vi "Create Indices.vi"(0 "Standard Engine Configuration":refnum<class "Standard Engine Configuration.lvclass">, 1 "Engine Tags":T1, 5 "main data dictionary":refnum<class "data dictionary.lvclass">, 7 "data description":T5, 9 "Module ID":string, 11 "error in":errorcluster) -> (4 "Input Transfer Specification":T2, 6 "Parameter Transfer Specifcation":T2, 8 "Result Transfer Specifcation":T2, 10 "Output Transfer Specifcation":T2, 15 "error out":errorcluster)   [LabVIEW 2013, in "Standard Engine Runtime.lvclass"]
doc: "Takes a single module's configuration and reformats that into a set of mappings."
uses:
  Standard Engine Runtime.lvclass
  <vilib>/NI/Tag Bus/dictionary/data dictionary.lvclass
  <vilib>/NI/Tag Bus Module Framework/channel/data tables.ctl
  <vilib>/NI/Tag Bus/dictionary table pair.ctl
  <vilib>/NI/Tag Bus/table/data table.ctl
  main engine/module method data.ctl
  <vilib>/NI/Tag Bus/table/transfer specification.ctl
  <vilib>/NI/Tag Bus/tag/Data Type.ctl
  Configuration/Standard Engine Configuration.lvclass
  <vilib>/NI/Module Execution Interface/Engine Configuration/engine configuration.lvclass
  <vilib>/NI/Tag Bus/tag/tag descriptor.lvclass
  <vilib>/NI/Tag Bus/table/data table.lvlib
  main engine/main engine.lvlib
  <vilib>/NI/Tag Bus Module Framework/channel/TBM channel.lvclass
  <vilib>/NI/Tag Bus/tag bus.lvlib
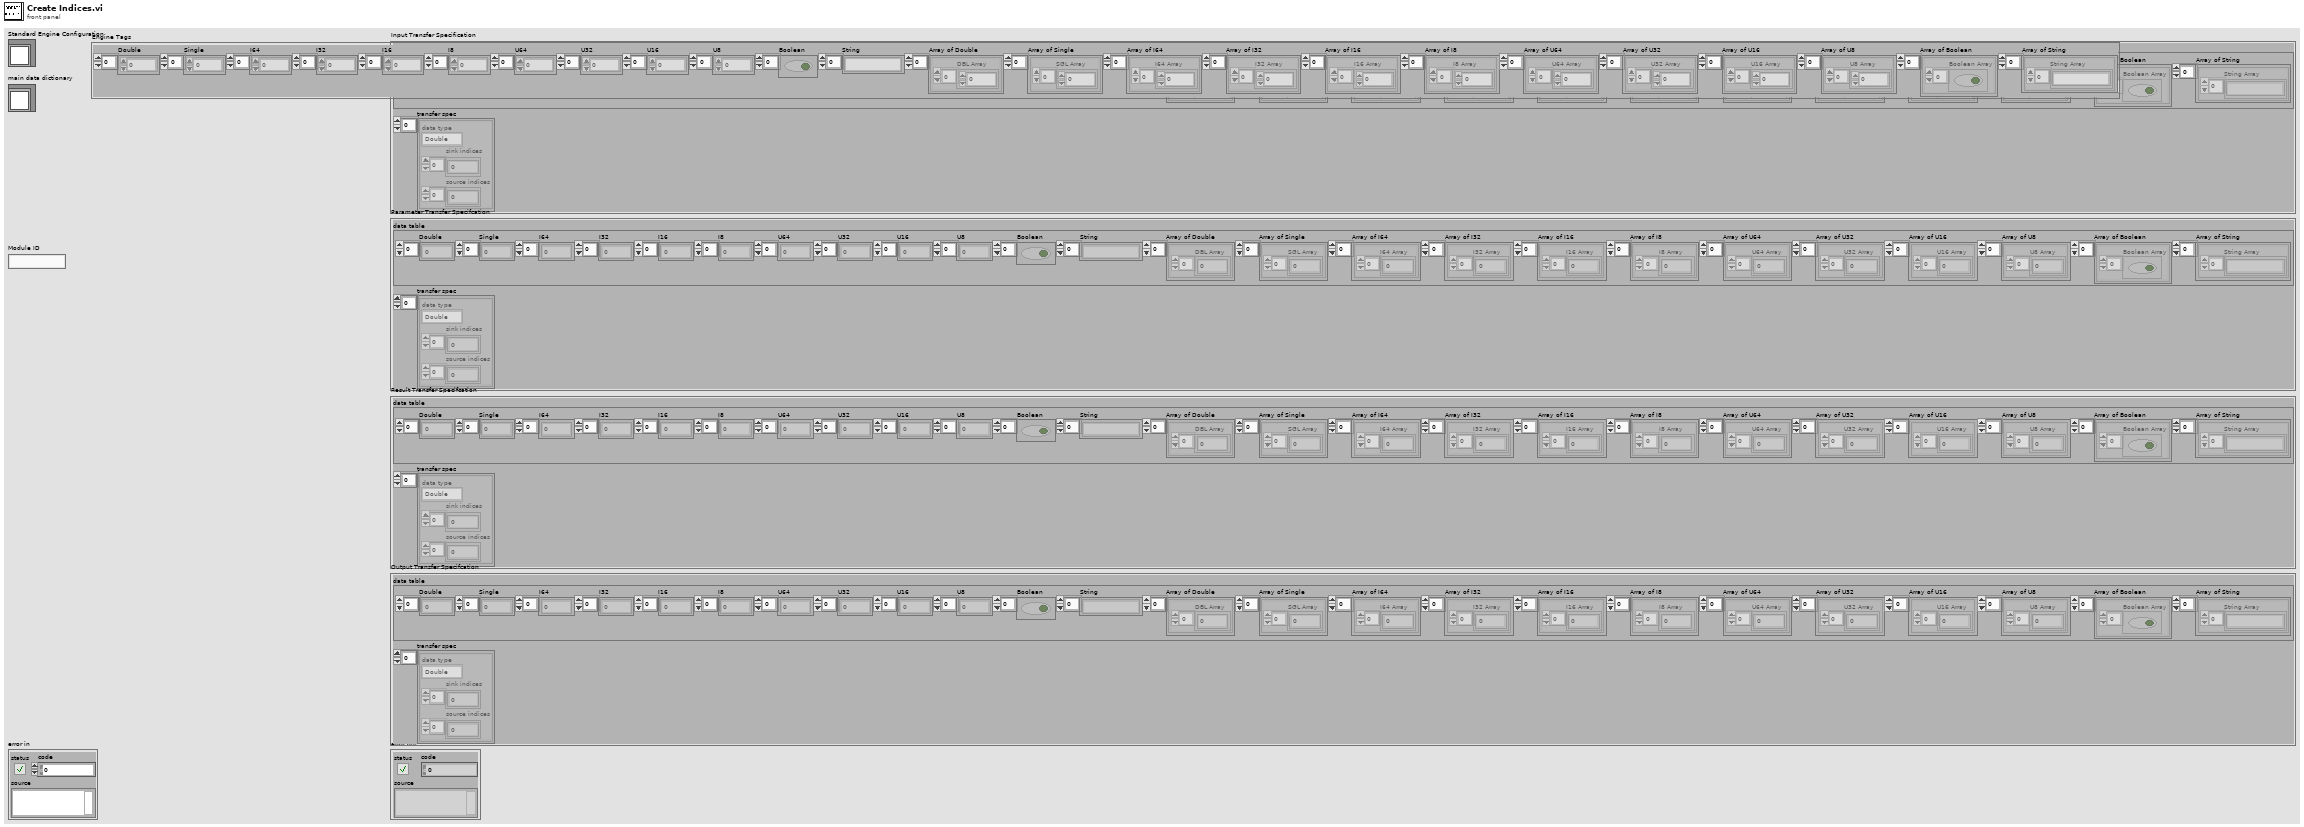
[diagram p1: front panel]
types:
  T1 = typedef "tag bus.lvlib/data table.lvlib/data table.ctl" = cluster{"Double":dbl[], "Single":sgl[], "I64":i64[], "I32":i32[], "I16":i16[], "I8":i8[], "U64":u64[], "U32":u32[], "U16":u16[], "U8":u8[], "Boolean":bool[], "String":string[], "Array of Double":cluster{"DBL Array":dbl[]}[], "Array of Single":cluster{"SGL Array":sgl[]}[], "Array of I64":cluster{"I64 Array":i64[]}[], "Array of I32":cluster{"I32 Array":i32[]}[], "Array of I16":cluster{"I16 Array":i16[]}[], "Array of I8":cluster{"I8 Array":i8[]}[], "Array of U64":cluster{"U64 Array":u64[]}[], "Array of U32":cluster{"U32 Array":u32[]}[], "Array of U16":cluster{"U16 Array":u16[]}[], "Array of U8":cluster{"U8 Array":u8[]}[], "Array of Boolean":cluster{"Boolean Array":bool[]}[], "Array of String":cluster{"String Array":string[]}[]}
  T2 = typedef "main engine.lvlib/module method data.ctl" = cluster{"data table":T1, "transfer spec":T3[]}
  T3 = typedef "tag bus.lvlib/data table.lvlib/transfer specification.ctl" = cluster{"data type":T4, "sink indices":i32[], "source indices":i32[]}
  T4 = typedef "tag bus.lvlib/tag descriptor.lvclass/Data Type.ctl" = enum16{"Double", "Single", "I64", "I32", "I16", "I8", "U64", "U32", "U16", "U8", "Boolean", "String", "Array of Double", "Array of Single", "Array of I64", "Array of I32", "Array of I16", "Array of I8", "Array of U64", "Array of U32", "Array of U16", "Array of U8", "Array of Boolean", "Array of String"}
  T5 = typedef "TBM channel.lvclass/data tables.ctl" = cluster{"input data":T6, "processing parameter":T6, "processing result":T6, "output data":T6}
  T6 = typedef "tag bus.lvlib/dictionary table pair.ctl" = cluster{"data dictionary":refnum<class "data dictionary.lvclass">, "data table":T1}
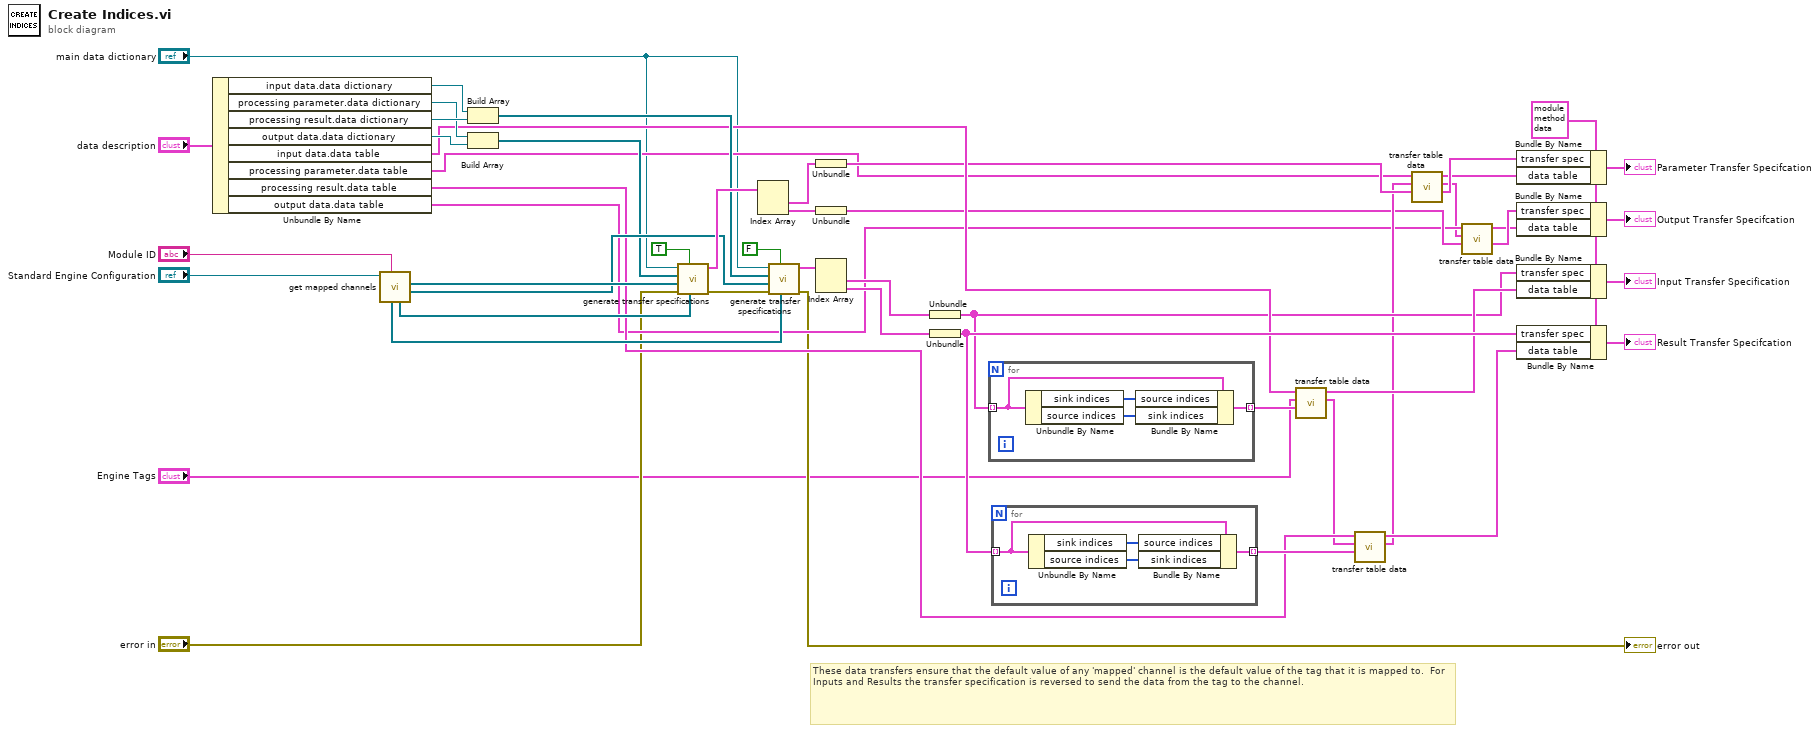
[diagram p0: block diagram]
diagram:
  w31 = T2 {"data table"={"Double"=[], "Single"=[], "I64"=[], "I32"=[], "I16"=[], "I8"=[], "U64"=[], "U32"=[], "U16"=[], "U8"=[], "Boolean"=[], "String"=[], "Array of Double"=[], "Array of Single"=[], "Array of I64"=[], "Array of I32"=[], "Array of I16"=[], "Array of I8"=[], "Array of U64"=[], "Array of U32"=[], "Array of U16"=[], "Array of U8"=[], "Array of Boolean"=[], "Array of String"=[]}, "transfer spec"=[]} ("method data")
  # "These data transfers ensure that the default value of any 'mapped' channel is the default value of the tag that it is mapped to.  For Inputs and Results the transfer specification is reversed to send the data from the tag to the channel."
  n1 = Unbundle By Name("data description") -> ("input data.data dictionary"=w37:refnum<class "data dictionary.lvclass">, "processing parameter.data dictionary"=w34:refnum<class "data dictionary.lvclass">, "processing result.data dictionary"=w36:refnum<class "data dictionary.lvclass">, "output data.data dictionary"=w33:refnum<class "data dictionary.lvclass">, "input data.data table"=w26:T1, "processing parameter.data table"=w19:T1, "processing result.data table"=w27:T1, "output data.data table"=w14:T1)
  n2 = call <vilib>:"get mapped channels.vi"("owner"="Module ID", "engine configuration in"="Standard Engine Configuration") -> ("write channels"=w42:refnum<class "TBM channel.lvclass">[], "read channels"=w50:refnum<class "TBM channel.lvclass">[], "paired read tag"=w39:refnum<class "tag descriptor.lvclass">[], "paired write tag"=w38:refnum<class "tag descriptor.lvclass">[])  [unwired: 5 in, 1 out]
  n3 = Build Array(w37, w36) -> (w35:refnum<class "data dictionary.lvclass">[])
  n4 = Build Array(w34, w33) -> (w32:refnum<class "data dictionary.lvclass">[])
  n5 = call "generate transfer specifications.vi"("paired tags"=w39, "main is source?"=TRUE, "error in"="error in", "channels"=w50, "dictionaries by class"=w32, "main data dictionary"="main data dictionary") -> ("error out"=w46:errorcluster, "transfer specifications"=w49:cluster{"transfer specification":T3[]}[])  [unwired: 4 in]
  n6 = Index Array(array=w49) -> (element #1=w48:cluster{"transfer specification":T3[]}, element #2=w47:cluster{"transfer specification":T3[]})  [unwired: 2 in]
  n7 = call "generate transfer specifications.vi"("paired tags"=w38, "main is source?"=FALSE, "error in"=w46, "channels"=w42, "dictionaries by class"=w35, "main data dictionary"="main data dictionary") -> ("error out"=→"error out":errorcluster, "transfer specifications"=w43:cluster{"transfer specification":T3[]}[])  [unwired: 4 in]
  n8 = Unbundle(w48) -> ("transfer specification"=w21:T3[])
  n9 = Unbundle(w47) -> ("transfer specification"=w16:T3[])
  n10 = Index Array(array=w43) -> (element #1=w44:cluster{"transfer specification":T3[]}, element #2=w45:cluster{"transfer specification":T3[]})  [unwired: 2 in]
  n11 = Unbundle(w44) -> ("transfer specification"=w22:T3[])
  n12 = Unbundle(w45) -> ("transfer specification"=w30:T3[])
  n13 = for {
    tunnel: w22 -> [w54] mode=indexing
    tunnel: [w51] -> w29 mode=indexing
    n14 = Unbundle By Name(w54) -> ("sink indices"=w53:i32[], "source indices"=w52:i32[])
    n15 = Bundle By Name(cluster=w54, "source indices"=w53, "sink indices"=w52) -> (w51:T3)
  }
  n16 = for {
    tunnel: w30 -> [w58] mode=indexing
    tunnel: [w55] -> w28 mode=indexing
    n17 = Unbundle By Name(w58) -> ("sink indices"=w57:i32[], "source indices"=w56:i32[])
    n18 = Bundle By Name(cluster=w58, "source indices"=w57, "sink indices"=w56) -> (w55:T3)
  }
  n19 = call <vilib>:"transfer table data.vi"("transfer specification in"=w29, "data table source in"="Engine Tags", "data table sink in"=w26) -> ("data table source out"=w23:T1, "data table sink out"=w25:T1)  [unwired: 6 in, 1 out]
  n20 = call <vilib>:"transfer table data.vi"("transfer specification in"=w28, "data table source in"=w23, "data table sink in"=w27) -> ("data table source out"=w17:T1, "data table sink out"=w24:T1)  [unwired: 6 in, 1 out]
  n21 = call <vilib>:"transfer table data.vi"("transfer specification in"=w21, "data table source in"=w17, "data table sink in"=w19) -> ("transfer specification out"=w20:T3[], "data table source out"=w12:T1, "data table sink out"=w18:T1)  [unwired: 6 in]
  n22 = call <vilib>:"transfer table data.vi"("transfer specification in"=w16, "data table source in"=w12, "data table sink in"=w14) -> ("transfer specification out"=w15:T3[], "data table sink out"=w13:T1)  [unwired: 6 in, 1 out]
  n23 = Bundle By Name(cluster=w31, "transfer spec"=w20, "data table"=w18) -> (→"Parameter Transfer Specifcation":T2)
  n24 = Bundle By Name(cluster=w31, "transfer spec"=w15, "data table"=w13) -> (→"Output Transfer Specifcation":T2)
  n25 = Bundle By Name(cluster=w31, "transfer spec"=w22, "data table"=w25) -> (→"Input Transfer Specification":T2)
  n26 = Bundle By Name(cluster=w31, "transfer spec"=w30, "data table"=w24) -> (→"Result Transfer Specifcation":T2)
